vi "direction.vi"(10 "upper limit":dbl, 11 "upper limit 2":dbl) -> (3 "Numeric":dbl)   [LabVIEW 2014]
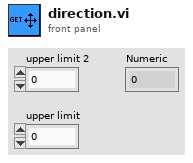
[diagram p1: front panel]
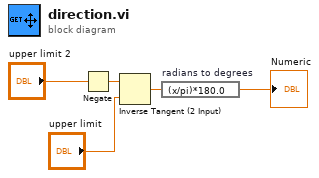
[diagram p0: block diagram]
diagram:
  n1 = Negate(x="upper limit 2") -> (-x=w2:dbl)
  n2 = Inverse Tangent (2 Input)(1:"upper limit", 2:w2) -> (0:w5:dbl)
  n3 = expression code="(x/pi)*180.0" "radians to degrees"(w5) -> (→"Numeric":dbl)
